vi "Bytes In Rune.vi"(11 "Byte":u8 format="%08b") -> (3 "Bytes in Rune":i8)   [LabVIEW 2019, in "JKI Unicode.lvlib" / "UTF-8 String.lvclass"]
doc: "JKI Unicode 1.0.0.7\nTomi Maila - JKI\nCopyright (c) 2016, JKI"
uses:
  UTF-8 String.lvclass
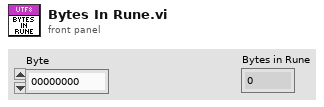
[diagram p1: front panel]
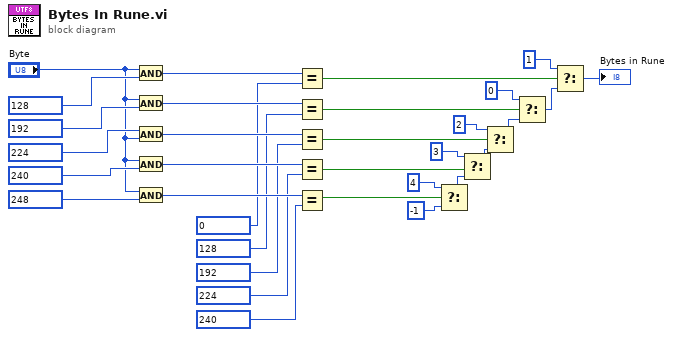
[diagram p0: block diagram]
diagram:
  n1 = And(x="Byte", y=u8 128 ("Byte")) -> (x .and. y?=w26:u8)
  n2 = And(x="Byte", y=u8 192 ("Byte")) -> (x .and. y?=w25:u8)
  n3 = And(x=u8 224 ("Byte"), y="Byte") -> (x .and. y?=w24:u8)
  n4 = And(x="Byte", y=u8 240 ("Byte")) -> (x .and. y?=w23:u8)
  n5 = And(x="Byte", y=u8 248 ("Byte")) -> (x .and. y?=w22:u8)
  n6 = Equal?(x=w26, y=u8 0 ("Byte")) -> (x = y?=w16:bool)
  n7 = Equal?(x=w25, y=u8 128 ("Byte")) -> (x = y?=w12:bool)
  n8 = Equal?(x=w24, y=u8 192 ("Byte")) -> (x = y?=w9:bool)
  n9 = Equal?(x=w23, y=u8 224 ("Byte")) -> (x = y?=w8:bool)
  n10 = Equal?(x=w22, y=u8 240 ("Byte")) -> (x = y?=w4:bool)
  n11 = Select(t=i8 4, s=w4, f=i8 -1) -> (s? t:f=w3:i8)
  n12 = Select(t=i8 3, s=w8, f=w3) -> (s? t:f=w6:i8)
  n13 = Select(t=i8 2, s=w9, f=w6) -> (s? t:f=w10:i8)
  n14 = Select(t=i8 0, s=w12, f=w10) -> (s? t:f=w13:i8)
  n15 = Select(t=i8 1, s=w16, f=w13) -> (s? t:f=→"Bytes in Rune":i8)
